vi "Sequence Check Drive RPM.vi"(10 "System State":map{string, dbl}(c390), 11 "Sequencer Data Context IN":T1={"Sequencer State"=enum."Idle", "Event Timeout"=-1, "Current Index"=0, "Sequence Timeout"=0, "Turbine RPM Array"=[], "Pump RPM Array"=[], "Duration (Seconds) Array"=[], "Folder Path"=path ""}) -> (3 "Sequencer Data Context OUT":T1={"Sequencer State"=enum."Idle", "Event Timeout"=-1, "Current Index"=0, "Sequence Timeout"=0, "Turbine RPM Array"=[], "Pump RPM Array"=[], "Duration (Seconds) Array"=[], "Folder Path"=path ""})   [LabVIEW 2024, in "Auto Modo.lvlib"]
uses:
  Auto Modo.lvlib
  Sequencer Data Context.ctl
  Sequencer State.ctl
  Logger/Logger.lvlib
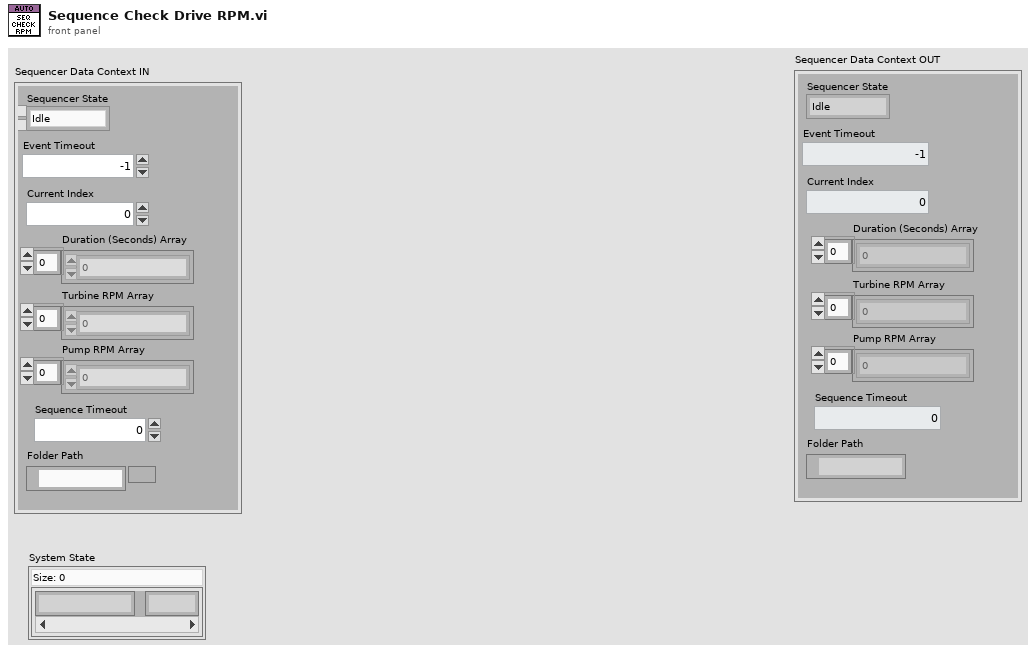
[diagram p1: front panel]
types:
  T1 = typedef "Auto Modo.lvlib/Sequencer Data Context.ctl" = cluster{"Sequencer State":T2, "Event Timeout":i32, "Current Index":i32, "Sequence Timeout":i32, "Turbine RPM Array":dbl[], "Pump RPM Array":dbl[], "Duration (Seconds) Array":dbl[], "Folder Path":path}
  T2 = typedef "Auto Modo.lvlib/Sequencer State.ctl" = enum16{"Idle", "Clear Drive Fault", "Check Drive Fault", "Set Ready to Switch ON", "Check Ready to Switch ON", "Enable Operation", "Check Enable Operation", "Set Drive RPM", "Check Drive RPM", "Next Drive RPM", "Final"}
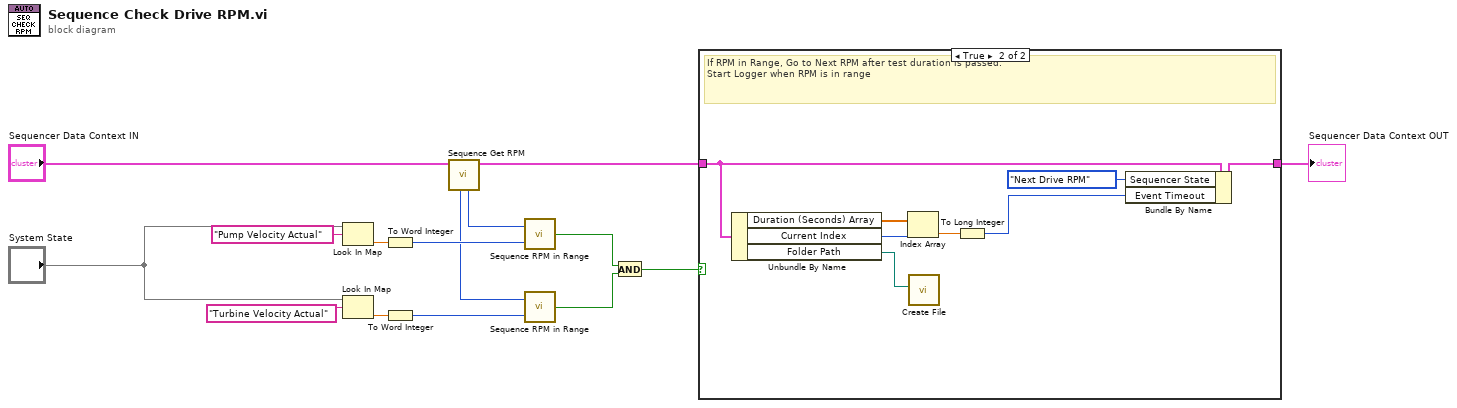
[diagram p0: block diagram]
diagram:
  n1 = Look In Map(map="System State", key="Pump Velocity Actual") -> (value=w10:dbl)  [unwired: 1 in, 1 out]
  n2 = Look In Map(map="System State", key="Turbine Velocity Actual") -> (value=w11:dbl)  [unwired: 1 in, 1 out]
  n3 = To Word Integer(number=w10) -> (16bit integer=w8:i16)
  n4 = To Word Integer(number=w11) -> (16bit integer=w9:i16)
  n5 = call "Sequence Get RPM.vi"("Sequencer Data Context IN"="Sequencer Data Context IN") -> ("Sequencer Data Context OUT"=w2:T1, "Pump RPM"=w7:i16, "Turbine RPM"=w6:i16)  [unwired: 8 in]
  n6 = call "Sequence RPM in Range.vi"("Actual RPM"=w8, "Target RPM"=w7) -> ("In Range?"=w5:bool)
  n7 = call "Sequence RPM in Range.vi"("Actual RPM"=w9, "Target RPM"=w6) -> ("In Range?"=w4:bool)
  n8 = And(x=w5, y=w4) -> (x .and. y?=w3:bool)
  n9 = case shown="True" w3 {
    tunnel: w2 -> [w16 w22]
    tunnel: [w16 w24] -> w1
    frame False {
      # "If not in range, keep waiting"
    }
    frame True {
      # "If RPM in Range, Go to Next RPM after test duration is passed. \nStart Logger when RPM is in range"
      n10 = Unbundle By Name(w22) -> ("Duration (Seconds) Array"=w21:dbl[], "Current Index"=w20:i32, "Folder Path"=w17:path)
      n11 = Index Array(array=w21, index=w20) -> (element=w19:dbl)
      n12 = call "Create File.vi"("Folder Path"=w17) -> ()  [unwired: 8 in, 3 out]
      n13 = To Long Integer(number=w19) -> (32bit integer=w18:i32)
      n14 = Bundle By Name(cluster=w22, "Sequencer State"=Sequencer_State."Next Drive RPM", "Event Timeout"=w18) -> (w24:T1)
    }
  }
  "Sequencer Data Context OUT" <- w1
